vi "TestingInterpolation.vi"() -> ()   [LabVIEW 2018]
uses:
  HistoryMeasurement.ctl
panel:
  out "XY Graph":cluster{u32[], dbl[]}[](graph)
  out "Interpolated Value":dbl
  out "Timestamp Key":u32
  in  "Interpolate Key":u32(slide) scale=0.0..1000.0
  out "s? t:f":T1[](array[typedef])
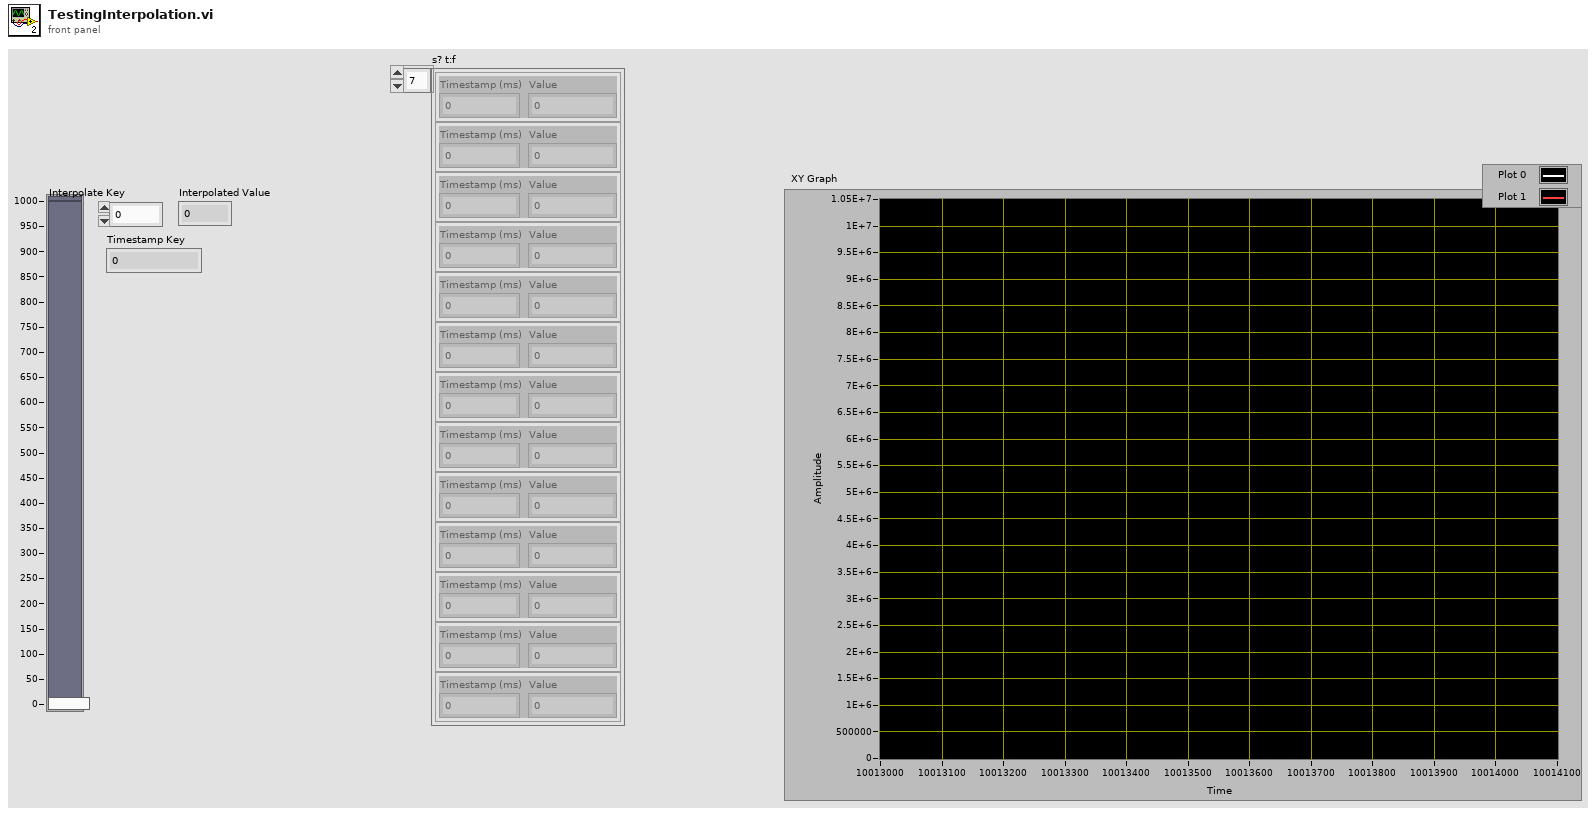
[diagram p1: front panel]
types:
  T1 = typedef "HistoryMeasurement.ctl" = cluster{"Timestamp (ms)":u32, "Value":dbl}
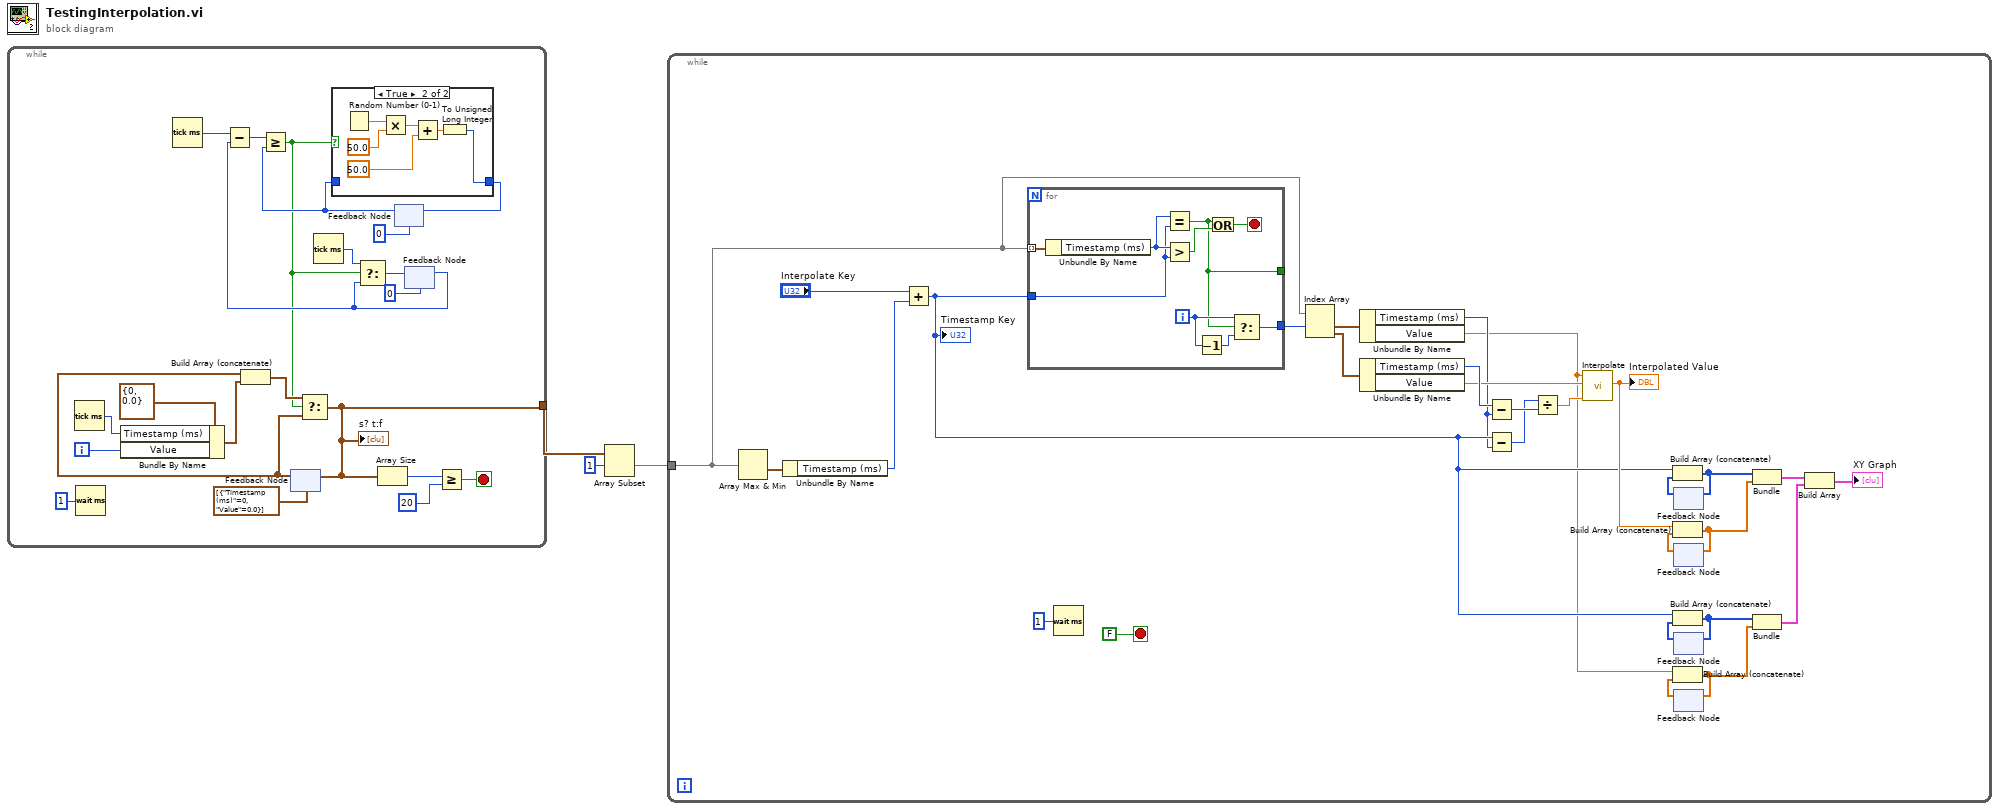
[diagram p0: block diagram]
diagram:
  n1 = while {
    tunnel: [w4] -> w2
    i -> [w11]
    stop <- w5 stop-if-true
    n2 = Tick Count (ms)() -> (millisecond timer value=w10:u32)
    n3 = Wait (ms)(milliseconds to wait=u32 1) -> ()  [unwired: 1 out]
    n4 = Bundle By Name(cluster=T1 {"Timestamp (ms)"=0, "Value"=0.0} ("Measurement"), "Timestamp (ms)"=w10, "Value"=w11) -> (w9:T1)
    n5 = Tick Count (ms)() -> (millisecond timer value=w22:u32)
    n6 = feedback #1(T1[] [{"Timestamp (ms)"=0, "Value"=0.0}]) -> (w14:T1[])
    n7 = Build Array (concatenate)(w14, w9) -> (w15:T1[])
    n8 = Tick Count (ms)() -> (millisecond timer value=w25:u32)
    n9 = feedback #2(u32 0) -> (w17:u32)
    n10 = feedback #3(u32 0 ("millisecond timer value")) -> (w21:u32)
    n11 = Subtract(x=w22, y=w21) -> (x-y=w20:u32)
    n12 = Greater Or Equal?(x=w20, y=w17) -> (x >= y?=w13:bool)
    n13 = Select(t=w15, s=w13, f=w14) -> (s? t:f=w4:T1[])
    "s? t:f" <- w4
    n14 = feedback-in #1(w4) -> ()
    n15 = case shown="True" w13 {
      tunnel: [w26 w27] -> w19
      tunnel: w17 -> [w26 _]
      frame False {
      }
      frame True {
        n16 = Random Number (0-1)() -> (number: 0 to 1=w32:dbl)
        n17 = Multiply(x=w32, y=50.0) -> (x*y=w30:dbl)
        n18 = Add(x=w30, y=50.0) -> (x+y=w28:dbl)
        n19 = To Unsigned Long Integer(number=w28) -> (unsigned 32bit integer=w27:u32)
      }
    }
    n20 = Select(t=w25, s=w13, f=w21) -> (s? t:f=w24:u32)
    n21 = Array Size(array=w4) -> (size(s)=w7:i32)
    n22 = feedback-in #2(w19) -> ()
    n23 = feedback-in #3(w24) -> ()
    n24 = Greater Or Equal?(x=w7, y=20) -> (x >= y?=w5:bool)
  }
  n25 = Array Subset(array=w2, index=1) -> (w3:T1[])  [unwired: 1 in]
  n26 = while {
    tunnel: w3 -> [w55]
    stop <- FALSE stop-if-true
    n27 = Array Max & Min(array=w55) -> (min value=w59:T1)  [unwired: 3 out]
    n28 = Unbundle By Name(w59) -> ("Timestamp (ms)"=w58:u32)
    n29 = Add(x="Interpolate Key", y=w58) -> (x+y=w41:u32)
    "Timestamp Key" <- w41
    n30 = for {
      tunnel: w55 -> [w70] mode=indexing
      tunnel: w41 -> [w68]
      tunnel: [w63] -> w56
      tunnel: [w62] -> _
      i -> [w64]
      stop <- w66 stop-if-true
      n31 = Unbundle By Name(w70) -> ("Timestamp (ms)"=w69:u32)
      n32 = Equal?(x=w69, y=w68) -> (x = y?=w62:bool)
      n33 = Greater?(x=w69, y=w68) -> (0:w67:bool)
      n34 = Decrement(x=w64) -> (x-1=w65:i32)
      n35 = Or(x=w62, y=w67) -> (x .or. y?=w66:bool)
      n36 = Select(t=w64, s=w62, f=w65) -> (s? t:f=w63:i32)
    }
    n37 = Wait (ms)(milliseconds to wait=u32 1) -> ()  [unwired: 1 out]
    n38 = Index Array(array=w55, index #1=w56) -> (element #1=w54:T1, element #2=w53:T1)  [unwired: 1 in]
    n39 = Unbundle By Name(w54) -> ("Timestamp (ms)"=w40:u32, "Value"=w34:dbl)
    n40 = Unbundle By Name(w53) -> ("Timestamp (ms)"=w49:u32, "Value"=w48:dbl)
    n41 = Subtract(x=w49, y=w40) -> (x-y=w52:u32)
    n42 = Subtract(x=w41, y=w40) -> (x-y=w51:u32)
    n43 = Divide(x=w51, y=w52) -> (x/y=w50:dbl)
    n44 = call "Interpolate.vi"("A (0 -1)"=w50, "High Value"=w48, "Low Value"=w34) -> ("Interolated Value"=w42:dbl)  [unwired: 8 in]
    "Interpolated Value" <- w42
    n45 = feedback #4() -> (w47:u32[])  [unwired: 1 in]
    n46 = Build Array (concatenate)(w41, w47) -> (w46:u32[])
    n47 = feedback-in #4(w46) -> ()
    n48 = feedback #5() -> (w45:dbl[])  [unwired: 1 in]
    n49 = Build Array (concatenate)(w42, w45) -> (w39:dbl[])
    n50 = feedback-in #5(w39) -> ()
    n51 = feedback #6() -> (w44:u32[])  [unwired: 1 in]
    n52 = Build Array (concatenate)(w41, w44) -> (w38:u32[])
    n53 = feedback-in #6(w38) -> ()
    n54 = feedback #7() -> (w43:dbl[])  [unwired: 1 in]
    n55 = Build Array (concatenate)(w34, w43) -> (w37:dbl[])
    n56 = feedback-in #7(w37) -> ()
    n57 = Bundle(w46, w39) -> (w36:cluster{u32[], dbl[]})  [unwired: 1 in]
    n58 = Bundle(w38, w37) -> (w33:cluster{u32[], dbl[]})  [unwired: 1 in]
    n59 = Build Array(w36, w33) -> (→"XY Graph":cluster{u32[], dbl[]}[])
  }
